vi "extract.vi"(8 "error in (no error)":errorcluster, 10 "VideoFile":refnum<class "VideoFile.lvclass">, 11 "CodecFactory in":refnum<class "CodecFactory.lvclass">) -> (0 "error out":errorcluster, 2 "Codec":refnum<class "Codec.lvclass">, 3 "CodecFactory out":refnum<class "CodecFactory.lvclass">)   [LabVIEW 2017, in "CodecFactory.lvclass"]
uses:
  CodecFactory.lvclass
  Codec Class/Codec.lvclass
  VideoFile Class/VideoFile.lvclass
  ConsoleOut/Print Options.ctl
  VideoFile Class/VideoFile.lvclass/VideoFile.ctl
  OggCompressionCodec Class/OggCompressionCodec.lvclass
  C:/Users/fflores/Documents/LabVIEW-Open-Projects/LabIVEW OOP Design Patterns/Facade Pattern/Codec Class/Codec.lvclass
  MPEG4CompressionCodec Class/MPEG4CompressionCodec.lvclass
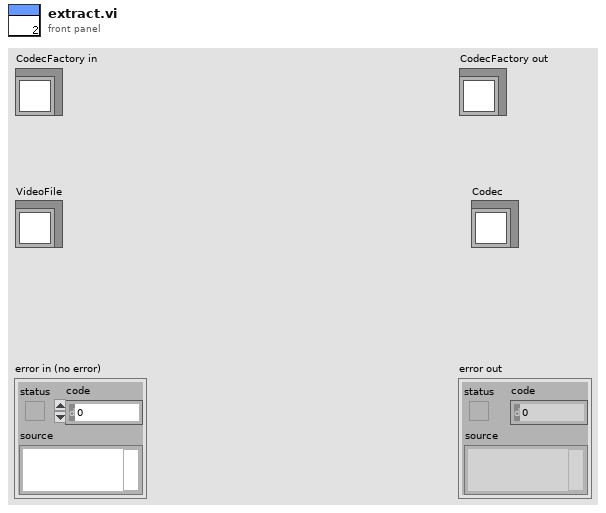
[diagram p1: front panel]
types:
  T1 = typedef "Print Options.ctl" = enum16{"Create", "Get Reference", "Print", "Print Header", "Close"}
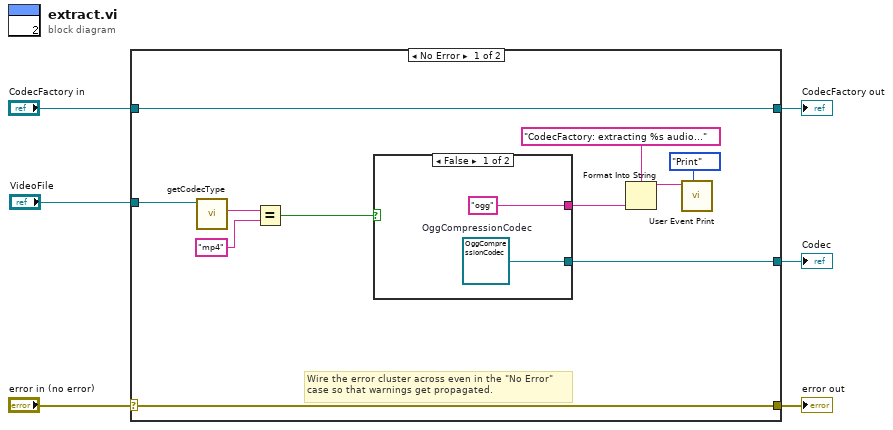
[diagram p0: block diagram]
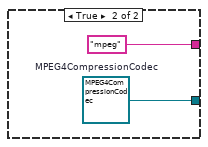
[diagram p2: hidden frame]
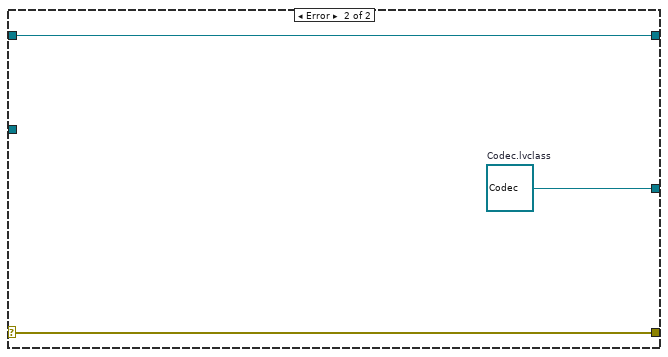
[diagram p3: hidden frame]
diagram:
  n1 = case shown="No Error" "error in (no error)" {
    selector: "error in (no error)" -> [w16 w24]
    tunnel: [w16 w24] -> w5
    tunnel: [w17 w23] -> w3
    tunnel: "CodecFactory in" -> [w17 w23]
    tunnel: "VideoFile" -> [w15 _]
    tunnel: [w11 w22] -> w1
    frame No Error {
      # "Wire the error cluster across even in the \"No Error\"\ncase so that warnings get propagated."
      n2 = call "getCodecType.vi"("VideoFile in"=w15) -> ("codecType"=w14:string)  [unwired: 8 in, 2 out]
      n3 = Equal?(x=w14, y="mp4") -> (x = y?=w12:bool)
      n4 = case shown="False" w12 {
        tunnel: [w19 w21] -> w11
        tunnel: ["ogg" ("y") "mpeg" ("y")] -> w10
        frame False {
          w19 = refnum<class "OggCompressionCodec.lvclass"> refnum  # OggCompressionCodec
        }
        frame True {
          w21 = refnum<class "MPEG4CompressionCodec.lvclass"> refnum  # MPEG4CompressionCodec
        }
      }
      n5 = Format Into String(format string="CodecFactory: extracting %s audio...", w10) -> (resulting string=w8:string)  [unwired: 2 in, 1 out]
      n6 = call "User Event Print.vi"("Options"=Print_Options."Print", "String to Print"=w8) -> ()  [unwired: 8 in, 2 out]
    }
    frame Error {
      w22 = refnum<class "Codec.lvclass"> refnum  # Codec.lvclass
    }
  }
  "error out" <- w5
  "CodecFactory out" <- w3
  "Codec" <- w1
